vi "Flush Msg Queue.vi"(8 "error in (no error)":errorcluster, 11 "Message Queue in":refnum<class "Delacor_lib_QMH_Message Queue.lvclass">) -> (0 "error out":errorcluster, 2 "Remaining States":string, 3 "Message Queue out":refnum<class "Delacor_lib_QMH_Message Queue.lvclass">)   [LabVIEW 2015, in "Tool Module.lvlib"]
uses:
  Tool Module.lvlib
  <vilib>/Delacor/Delacor QMH/Libraries/Message Queue_class/Delacor_lib_QMH_Message Queue.lvclass
  <vilib>/Delacor/Delacor QMH/Libraries/Message Queue_class/Delacor_lib_QMH_Message Queue.lvclass/Delacor_lib_QMH_Message Queue.ctl
  <vilib>/Delacor/Delacor QMH/Libraries/Message Queue_class/Delacor_lib_QMH_Enqueue Message (Single).vi
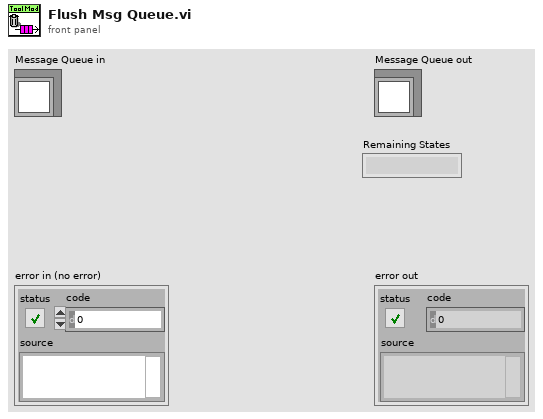
[diagram p1: front panel]
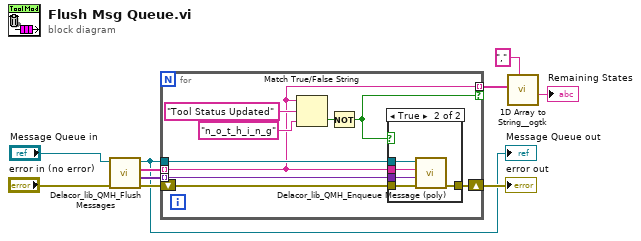
[diagram p0: block diagram]
diagram:
  n1 = call-dynamic "Delacor_lib_QMH_Flush Messages.vi"("error in (no error)"="error in (no error)", "Message Queue in"="Message Queue in") -> ("error out"=w6:errorcluster, "Remaining Message Data"=w7:variant[], "Remaining Messages"=w8:string[], "Message Queue out"=w4:refnum<class "Delacor_lib_QMH_Message Queue.lvclass">)  [unwired: 6 in]
  "Message Queue out" <- w4
  n2 = for {
    tunnel: w8 -> [w11] mode=indexing
    tunnel: w7 -> [w14] mode=indexing
    tunnel: [w11] -> w3 mode=indexing if=w12
    tunnel: w4 -> [w13]
    shift-right: [w15] -> w5
    shift-left: w6 -> [w16]
    n3 = Match True/False String(2:"n_o_t_h_i_n_g" ("false string"), 3:"Tool Status Updated", 4:w11) -> (0:w17:bool)  [unwired: 1 out]
    n4 = Not(x=w17) -> (.not. x?=w12:bool)
    n5 = case shown="True" w12 {
      tunnel: w16 -> [w20 w25]
      tunnel: [w20 w24] -> w15
      tunnel: w14 -> [_ w23]
      tunnel: w13 -> [_ w22]
      tunnel: w11 -> [_ w21]
      frame False {
      }
      frame True {
        n6 = call-poly <vilib>:"Delacor_lib_QMH_Enqueue Message (poly).vi"("error in (no error)"=w25, "Message Data"=w23, "Message"=w21, "Message Queue in"=w22) -> ("error out"=w24:errorcluster)  [unwired: 6 in, 1 out]
      }
    }
  }
  "error out" <- w5
  n7 = call <userlib>:"1D Array to String__ogtk.vi"("delimiter (Tab)"=",", "Array of Strings"=w3) -> ("delimited string"=→"Remaining States":string)  [unwired: 9 in]
